vi "_020.vi"() -> ()   [LabVIEW 2024]
panel:
  in  "OK Button 3":bool
  in  "OK Button 2":bool
  in  "OK Button 1":bool
  out "Iteration":i32
  in  "Horizontal Fill Slide 2":dbl(slide) scale=0.0..10.0
  in  "stop":bool
  out "Gauge":dbl(knob) scale=0.0..10.0
  in  "Horizontal Fill Slide":dbl(slide) scale=0.0..10.0
  # "To make a normal oprn without using Event Structure :"
  # "Poling"
  # "(Disadvantages)"
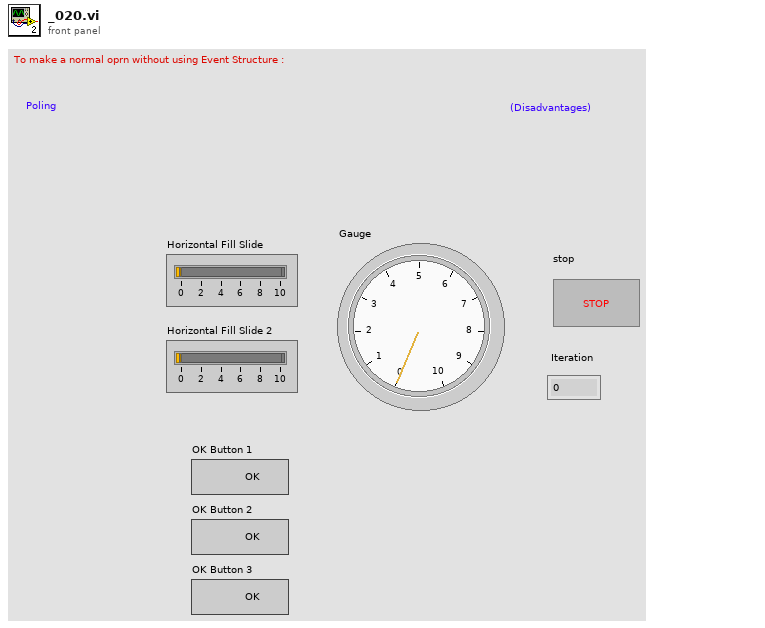
[diagram p1: front panel]
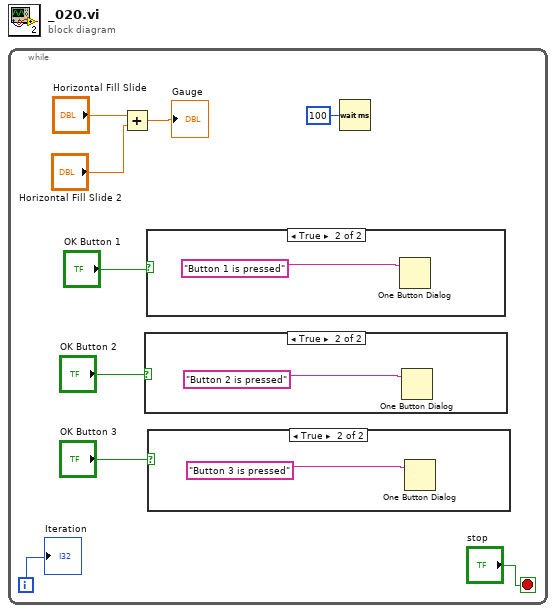
[diagram p0: block diagram]
diagram:
  n1 = while {
    i -> [w4]
    stop <- "stop" stop-if-true
    n2 = Add(x="Horizontal Fill Slide", y="Horizontal Fill Slide 2") -> (x+y=→"Gauge":dbl)
    n3 = case shown="True" "OK Button 2" {
      frame False {
      }
      frame True {
        n4 = One Button Dialog(message="Button 2 is pressed") -> ()  [unwired: 1 in, 1 out]
      }
    }
    n5 = case shown="True" "OK Button 1" {
      frame False {
      }
      frame True {
        n6 = One Button Dialog(message="Button 1 is pressed") -> ()  [unwired: 1 in, 1 out]
      }
    }
    n7 = case shown="True" "OK Button 3" {
      frame False {
      }
      frame True {
        n8 = One Button Dialog(message="Button 3 is pressed") -> ()  [unwired: 1 in, 1 out]
      }
    }
    n9 = Wait (ms)(milliseconds to wait=u32 100) -> ()  [unwired: 1 out]
    "Iteration" <- w4
  }
